vi "临界安全监督实测.vi"() -> ()   [LabVIEW 2020]
uses:
  <vilib>/Utility/sysdir.llb/System Directory Type.ctl
  <vilib>/Utility/error.llb/DialogType.ctl
  <vilib>/Utility/miscctls.llb/LVRowAndColumnTypeDef.ctl
  <vilib>/Analysis/baseanly.llb/Mean (DBL).vi
  GlobalVariable.vi
  <vilib>/Utility/inputDevices.llb/mouseAcquire.vi
  <vilib>/Analysis/NI_AALBase.lvlib
panel:
  in  "操作选项卡":enum32{"数据记录", "监督设置"}(tab)
  out "Table":string[][](table) caption="汇总表格"
  out "表象周期":sgl[](array[numeric])
  out "中子通量":sgl[](array[numeric])
  in  "保存表格":bool
  in  "添加记录":bool
  in  "显示临界曲线":bool
  in  "重设间隔":i32(knob)=1 min=1 max=100 step=1 scale=1.0..100.0
  in  "周期拟合个数":i32(knob)=1 min=1 max=100 step=1 scale=1.0..100.0
  out "堆芯参数：":dbl
  in  "堆芯参数项":u16(ring) items=["S棒位"]
  out "数选个数":i32
  in  "停止监督":bool
  in  "输入备注说明":string
  out "曲线5数字":dbl
  out "曲线4数字":dbl caption="D棒位"
  out "曲线3数字":dbl caption="电流2a周期"
  out "曲线2数字":dbl caption="电流2a"
  out "曲线1数字":dbl caption="电流1a周期"
  out "曲线0数字":dbl caption="电流1a"
  in  "自动/手动调整X标尺？":bool
  in  "X标尺最小-":bool
  in  "X标尺最小+":bool
  in  "自动调整Y标尺？":bool
  in  "Y标尺最小-":bool
  in  "Y标尺最小+":bool
  in  "Y标尺最大-":bool
  in  "Y标尺最大+":bool
  in  "曲线开关4":bool=TRUE
  in  "曲线开关5":bool=TRUE
  in  "曲线开关3":bool=TRUE
  in  "曲线开关2":bool=TRUE
  in  "曲线开关1":bool=TRUE
  in  "曲线开关0":bool=TRUE
  out "GraphChart":dbl[][](graph)
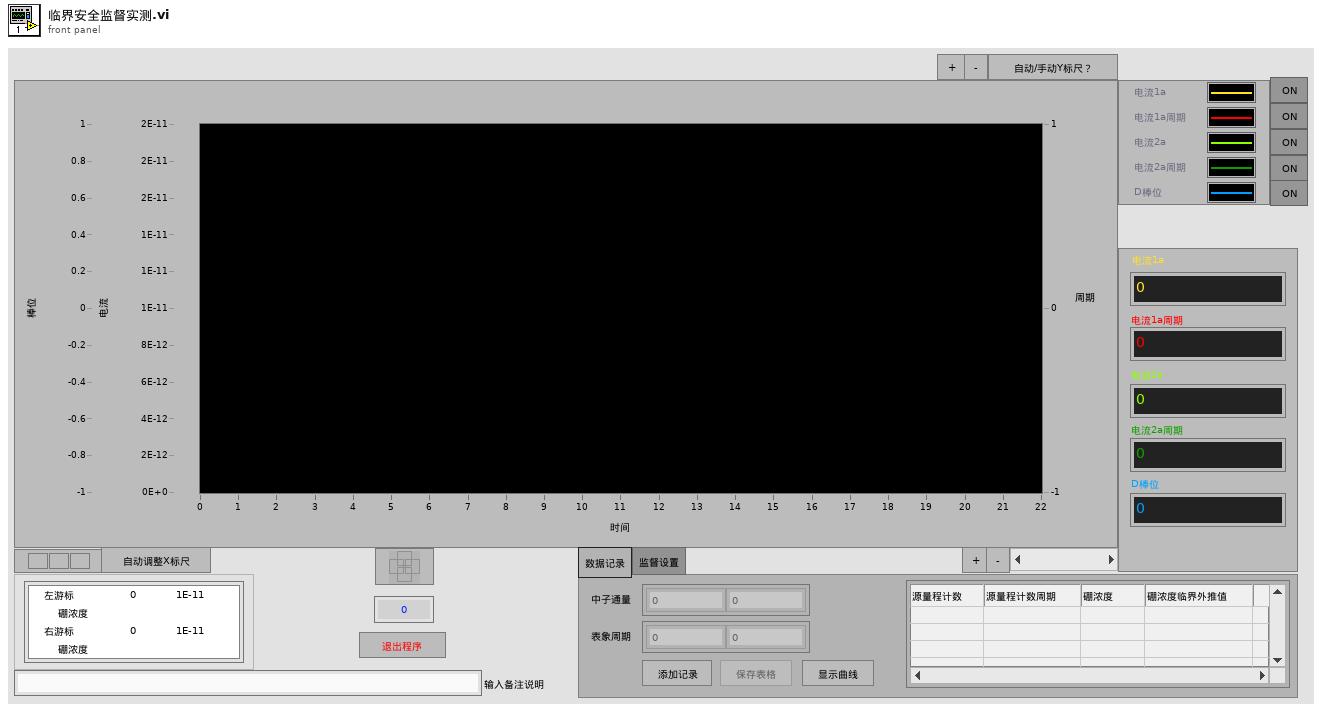
[diagram p1: front panel]
types:
  T1 = enum16{"open", "open or create", "create or replace", "create", "open (read only)"}
  T2 = typedef "System Directory Type.ctl" = i32
  T3 = typedef "DialogType.ctl" = u16
  T4 = enum8{"Enabled", "Disabled", "Disabled and Grayed Out"}
  T5 = enum16{"open", "replace", "create", "open or create", "replace or create", "replace or create with confirmation"}
  T6 = typedef "LVRowAndColumnTypeDef.ctl" = cluster{"Row":i32, "Column":i32}
  T7 = typedef "LVCursorListTypeDef.ctl" = cluster{"Name":string, "Color":u32, "Style":u8, "Point Style":u8, "Name Visible":bool, "Allow Drag":bool, "Cursor Mode":u32, "Plot":i32, "Index":i32, "Position":cluster{"X":dbl, "Y":dbl}, "X Scale":u32, "Y Scale":u32, "Watch Plots":i32[], "Watch All Plots":bool, "Plot Area":i32, "Label Offset":cluster{"X":dbl, "Y":dbl}}[]
  T8 = cluster{"Name":string, "Color":u32, "Style":u8, "Point Style":u8, "Name Visible":bool, "Allow Drag":bool, "Cursor Mode":u32, "Plot":i32, "Index":i32, "Position":cluster{"X":dbl, "Y":dbl}, "X Scale":u32, "Y Scale":u32, "Watch Plots":i32[], "Watch All Plots":bool, "Plot Area":i32, "Label Offset":cluster{"X":dbl, "Y":dbl}}
  T9 = cluster{"button 1":bool, "button 2":bool, "button 3":bool, "button 4":bool}
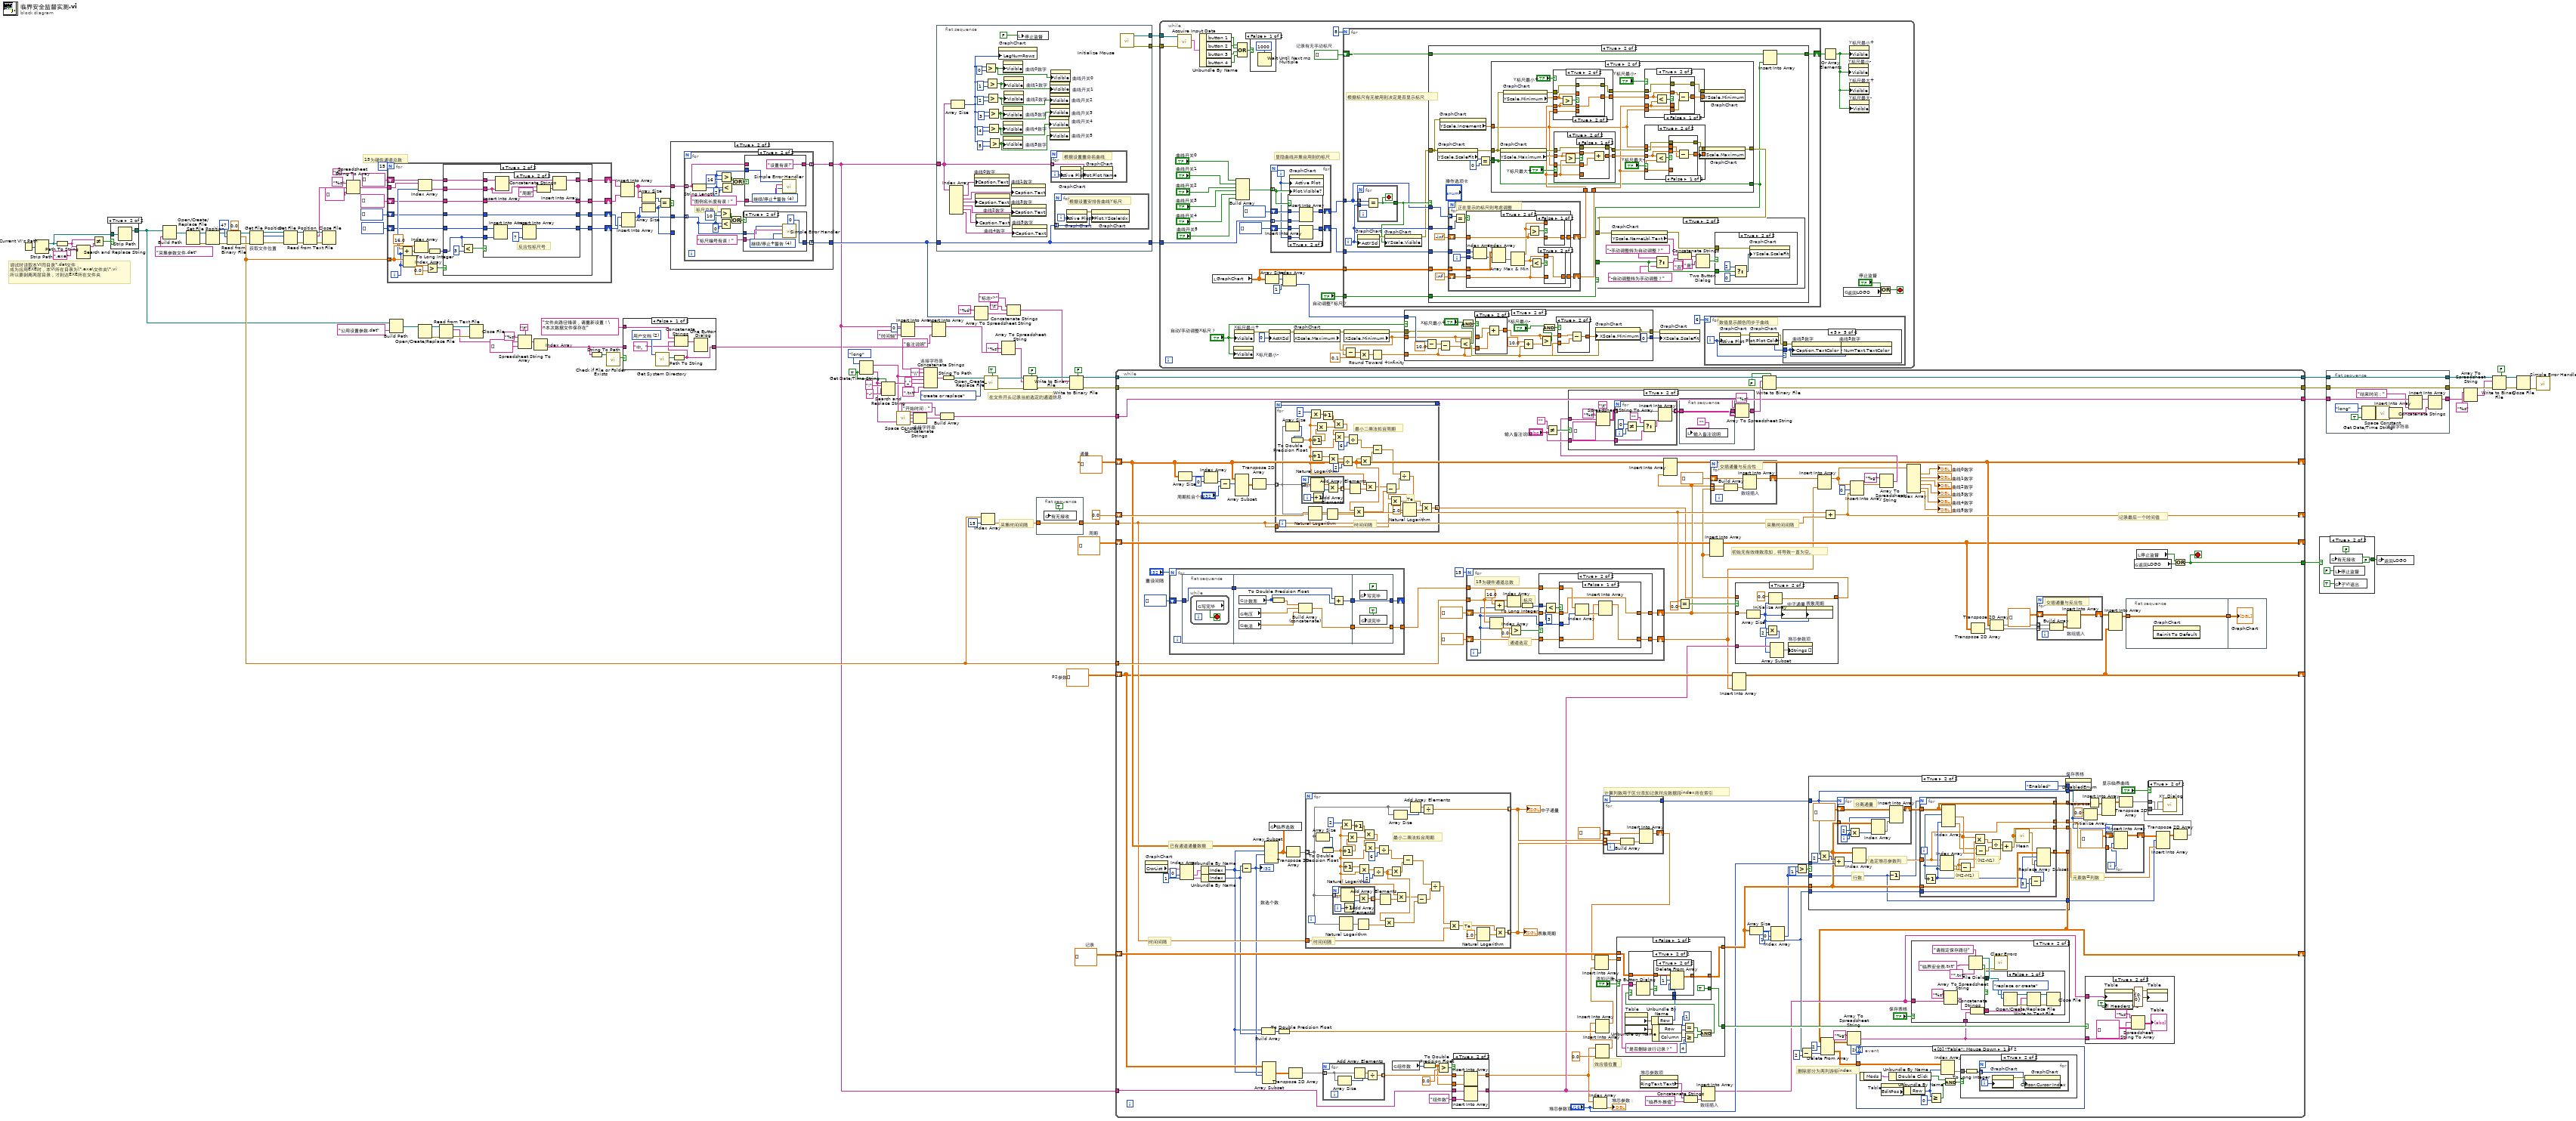
[diagram p0: block diagram]
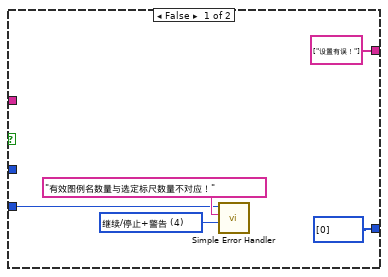
[diagram p4: hidden frame]
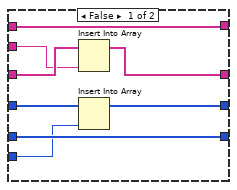
[diagram p8: hidden frame]
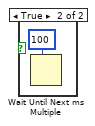
[diagram p9: hidden frame]
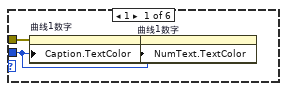
[diagram p10: hidden frame]
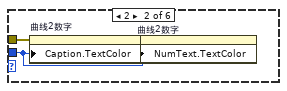
[diagram p11: hidden frame]
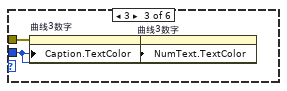
[diagram p12: hidden frame]
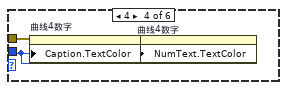
[diagram p13: hidden frame]
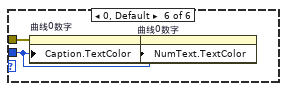
[diagram p14: hidden frame]
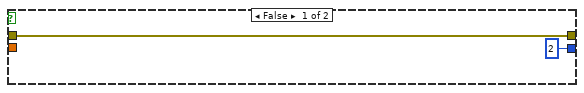
[diagram p15: hidden frame]
diagram:
  w22 = dbl[][] []  # P2参数
  w23 = dbl[][] []  # 周期
  w24 = dbl[][] []  # 通量
  w25 = dbl[][] []  # 记录
  w53 = TRUE ("需要秒？(F)")
  # "采集时间间隔"
  # "调试时读取本VI同目录*.dat文件，\n成为应用EXE时，本VI所在目录为\\*.exe\\文件夹\\*.vi\n所以要剥离两层目录，才到达EXE所在文件夹"
  # "15为硬件通道总数"
  # "在文件开头记录当前选定的通道信息"
  n1 = Current VI's Path() -> (path=w36:path)
  n2 = Strip Path(path=w36) -> (stripped path=w31:path)  [unwired: 1 out]
  n3 = Path To String(path=w31) -> (string=w33:string)
  n4 = Search and Replace String(input string=w33, search string=".exe" ("搜索字符串")) -> (result string=w34:string)  [unwired: 6 in, 3 out]
  n5 = Not Equal?(x=w33, y=w34) -> (x != y?=w32:bool)
  n6 = case shown="True" w32 {
    tunnel: w31 -> [w126 w128]
    tunnel: [w126 w127] -> w9
    frame False {
    }
    frame True {
      n7 = Strip Path(path=w128) -> (stripped path=w127:path)  [unwired: 1 out]
    }
  }
  n8 = Build Path(base path=w9, name or relative path="采集参数文件.dat") -> (appended path=w102:path)
  n9 = Open/Create/Replace File(file path (use dialog)=w102) -> (refnum out=w99:refnum<file>, error out=w98:errorcluster)  [unwired: 5 in, 1 out]
  n10 = Set File Position(refnum=w99, error in=w98) -> (refnum out=w97:refnum<file>, error out=w96:errorcluster)  [unwired: 2 in]
  n11 = Read from Binary File(5:sgl 0.0 ("byte stream type"), 8:w96, 10:47 ("count"), 11:w97) -> (0:w100:errorcluster, 2:w30:sgl[], 3:w101:refnum<file>)  [unwired: 2 in, 1 out]
  n12 = Get File Position "获取文件位置"(4:w100, 7:w101) -> (0:w104:errorcluster, 2:w91:i64, 3:w105:refnum<file>)
  n13 = Set File Position(offset (in bytes) (0)=w91, refnum=w105, error in=w104) -> (refnum out=w95:refnum<file>, error out=w94:errorcluster)  [unwired: 1 in]
  n14 = Read from Text File(file (use dialog)=w95, error in=w94) -> (refnum out=w92:refnum<file>, text=w87:string, error out=w93:errorcluster)  [unwired: 1 in, 2 out]
  n15 = Close File(refnum=w92, error in=w93) -> ()  [unwired: 2 out]
  n16 = Spreadsheet String To Array(delimiter (Tab)="\t", format string="%s", spreadsheet string=w87, array type (2D Dbl)=string[] [] ("添加的数组")) -> (array=w86:string[])
  n17 = for {
    N: 15 -> [_]
    tunnel: w30 -> [w140]
    tunnel: w86 -> [w147]
    shift-right: [w144] -> w80
    shift-left: string[] [] ("添加的数组") -> [w143]
    shift-right: [w135] -> w78
    shift-left: i32[] [] ("添加的数组") -> [w136]
    shift-right: [w133] -> w79
    shift-left: string[] [] ("添加的数组") -> [w134]
    shift-right: [w131] -> w77
    shift-left: i32[] [] ("添加的数组") -> [w132]
    i -> [w137]
    n18 = Add(x=16.0, y=w137) -> (x+y=w139:dbl)
    n19 = Index Array(array=w140, index=w137) -> (element=w146:sgl)
    n20 = Index Array(array=w140, index=w139) -> (element=w130:sgl)
    n21 = Index Array(array=w147, index=w137) -> (element=w141:string)
    n22 = Greater?(x=w146, y=sgl 0.0) -> (0:w142:bool)
    n23 = To Long Integer(number=w130) -> (32bit integer=w129:i32)
    n24 = case shown="True" w142 {
      tunnel: [w151 w163] -> w144
      tunnel: w143 -> [w151 w159]
      tunnel: w141 -> [_ w158]
      tunnel: [w150 w161] -> w135
      tunnel: w136 -> [w150 w153]
      tunnel: w134 -> [w149 w157]
      tunnel: [w149 w156] -> w133
      tunnel: w132 -> [w148 w155]
      tunnel: [w148 w154] -> w131
      tunnel: w129 -> [_ w152]
      frame False {
      }
      frame True {
        n25 = Less?(x=w152, y=3) -> (x < y?=w160:bool)
        n26 = case shown="True" w160 {
          tunnel: w159 -> [w170 w179]
          tunnel: [w170 w184] -> w163
          tunnel: w153 -> [w171 w174]
          tunnel: [w171 w183] -> w161
          tunnel: w158 -> [w167 w177]
          tunnel: w157 -> [w169 w176]
          tunnel: [w168 w176] -> w156
          tunnel: [w164 w175] -> w154
          tunnel: w155 -> [w166 w175]
          tunnel: w152 -> [w165 w172]
          frame False {
            n27 = Insert Into Array(array=w169, new element=w167) -> (w168:string[])  [unwired: 1 in]
            n28 = Insert Into Array(array=w166, new element=w165) -> (w164:i32[])  [unwired: 1 in]
          }
          frame True {
            # "反应性标尺号"
            n29 = Insert Into Array(array=w174, new element=w172) -> (w173:i32[])  [unwired: 1 in]
            n30 = Insert Into Array(array=w179, new element=w177) -> (w178:string[])  [unwired: 1 in]
            n31 = Insert Into Array(array=w173, new element=7 ("新元素/子数组")) -> (w183:i32[])  [unwired: 1 in]
            n32 = Concatenate Strings(w177, "周期" ("字符串")) -> (w181:string)
            n33 = Insert Into Array(array=w178, new element=w181) -> (w184:string[])  [unwired: 1 in]
          }
        }
      }
    }
  }
  n34 = Build Path(base path=w9, name or relative path="公用设置参数.dat") -> (appended path=w19:path)
  n35 = Open/Create/Replace File(file path (use dialog)=w19) -> (refnum out=w16:refnum<file>, error out=w15:errorcluster)  [unwired: 5 in, 1 out]
  n36 = Read from Text File(file (use dialog)=w16, error in=w15) -> (refnum out=w17:refnum<file>, text=w11:string, error out=w18:errorcluster)  [unwired: 1 in, 2 out]
  n37 = Close File(refnum=w17, error in=w18) -> ()  [unwired: 2 out]
  n38 = Spreadsheet String To Array(delimiter (Tab)="\t", format string="%s", spreadsheet string=w11, array type (2D Dbl)=string[] [] ("添加的数组")) -> (array=w10:string[])
  n39 = Index Array(array=w10) -> (element=w3:string)  [unwired: 1 in]
  n40 = String To Path(string=w3) -> (path=w5:path)
  n41 = call <vilib>:"Check if File or Folder Exists.vi"("path"=w5) -> ("file or folder exists?"=w4:bool)  [unwired: 8 in, 2 out]
  n42 = Insert Into Array(array=w80, new element=w79) -> (w72:string[])  [unwired: 1 in]
  n43 = Insert Into Array(array=w78, new element=w77) -> (w73:i32[])  [unwired: 1 in]
  n44 = case shown="False" w4 {
    tunnel: w3 -> [_ w191]
    tunnel: [w185 w191] -> w2
    tunnel: "文件夹路径错误，请重新设置！\n本次数据文件保存在" ("消息") -> [w189 _]
    frame False {
      w190 = T2 2 items=["用户目录"=0, "用户桌面"=1, "用户文档"=2, "用户应用程序数据"=3, "用户设置"=4, "用户临时目录"=5, "公共文档"=6, "公共应用程序数据"=7, "公共设置"=8, "公共缓存"=13, "系统核心库"=9, "系统安装库"=10, "应用程序文件"=11, "启动盘根目录"=12] ("system directory type")
      n45 = call <vilib>:"Get System Directory.vi"("system directory type"=w190) -> ("system directory"=w187:path)  [unwired: 10 in]
      n46 = Path To String(path=w187) -> (string=w185:string)
      n47 = Concatenate Strings(w189, w185, "中。" ("字符串")) -> (w188:string)
      n48 = One Button Dialog(message=w188) -> ()  [unwired: 1 in, 1 out]
    }
    frame True {
    }
  }
  n49 = Array Size(array=w72) -> (size(s)=w76:i32)
  n50 = Array Size(array=w73) -> (size(s)=w74:i32)
  n51 = Equal?(x=w76, y=w74) -> (x = y?=w75:bool)
  n52 = case shown="True" w75 {
    tunnel: w74 -> [w194 _]
    tunnel: w73 -> [_ w200]
    tunnel: w72 -> [_ w199]
    tunnel: [i32[] [0] w198] -> w63
    tunnel: [string[] ["设置有误！"] w197] -> w26
    frame False {
      w196 = T3 4 items=["无对话框", "确定信息", "继续或停止信息", "确定信息＋警告", "继续/停止+警告"] ("type of dialog (OK msg:1)")
      n53 = call <vilib>:"Simple Error Handler.vi"("error code (no error:0)"=w194, "error source (\" \")"="有效图例名数量与选定标尺数量不对应！" ("error source (\" \")"), "type of dialog (OK msg:1)"=w196) -> ()  [unwired: 2 in, 5 out]
    }
    frame True {
      n54 = for {
        tunnel: w200 -> [w205] mode=indexing
        tunnel: w199 -> [w202] mode=indexing
        tunnel: [w203] -> w198 mode=indexing
        tunnel: [w201] -> w197 mode=indexing
        # "标尺总数"
        n55 = String Length(string=w202) -> (length=w207:i32)
        n56 = Greater?(x=w205, y=10) -> (0:w210:bool)
        n57 = Less?(x=w205, y=0) -> (x < y?=w209:bool)
        n58 = Greater?(x=w207, y=16) -> (0:w214:bool)
        n59 = Less?(x=w207, y=2) -> (x < y?=w215:bool)
        n60 = Or(x=w210, y=w209) -> (x .or. y?=w206:bool)
        n61 = Or(x=w214, y=w215) -> (x .or. y?=w213:bool)
        n62 = case shown="True" w206 {
          tunnel: "标尺编号有误！" ("error source (\" \")") -> [_ w222]
          tunnel: w205 -> [w218 w221]
          tunnel: [w218 0] -> w203
          frame False {
          }
          frame True {
            w220 = T3 4 items=["无对话框", "确定信息", "继续或停止信息", "确定信息＋警告", "继续/停止+警告"] ("type of dialog (OK msg:1)")
            n63 = call <vilib>:"Simple Error Handler.vi"("error code (no error:0)"=w221, "error source (\" \")"=w222, "type of dialog (OK msg:1)"=w220) -> ()  [unwired: 2 in, 5 out]
          }
        }
        n64 = case shown="True" w213 {
          tunnel: "图例名长度有误！" ("error source (\" \")") -> [_ w227]
          tunnel: w207 -> [_ w226]
          tunnel: w202 -> [w223 _]
          tunnel: [w223 "设置有误!"] -> w201
          frame False {
          }
          frame True {
            w225 = T3 4 items=["无对话框", "确定信息", "继续或停止信息", "确定信息＋警告", "继续/停止+警告"] ("type of dialog (OK msg:1)")
            n65 = call <vilib>:"Simple Error Handler.vi"("error code (no error:0)"=w226, "error source (\" \")"=w227, "type of dialog (OK msg:1)"=w225) -> ()  [unwired: 2 in, 5 out]
          }
        }
      }
    }
  }
  n66 = Get Date/Time String(date format (0)=enum16{"short", "long", "abbreviated"}."long" ("日期格式(0)"), want seconds? (F)=w53) -> (date string=w51:string, time string=w50:string)  [unwired: 1 in]
  n67 = Search and Replace String(replace all?=w53, input string=w50, search string=":", replace string="-" ("replace string (\"\")")) -> (result string=w121:string)  [unwired: 4 in, 3 out]
  n68 = call <vilib>:"Space Constant.vi"() -> ("String"=w52:string)
  n69 = Insert Into Array(array=w26, index=0 ("索引"), new element="时间轴" ("新元素/子数组")) -> (w57:string[])
  n70 = Concatenate Strings "连接字符串"(w51, w52, w50) -> (w47:string)
  n71 = Concatenate Strings "连接字符串"(w2, "\\" ("字符串"), w51, "_" ("string"), w121, ".txt" ("string")) -> (w7:string)
  n72 = Insert Into Array(array=w57, new element="备注说明" ("新元素/子数组")) -> (w56:string[])  [unwired: 1 in]
  n73 = flat-sequence {
    tunnel: w26 -> [w239]
    tunnel: [w229] -> w111
    tunnel: w63 -> [w229]
    tunnel: [w231] -> w109
    tunnel: [w230] -> w108
    frame #0 {
      n74 = Index Array(array=w239) -> (element #1=w251:string, element #2=w250:string, element #3=w249:string, element #4=w248:string, element #5=w247:string, element #6=w246:string)  [unwired: 6 in]
      n75 = Array Size(array=w239) -> (size(s)=w232:i32)
      n76 = property on="曲线0数字" class="DigNum (strict)"("Caption.Text"=w251) -> ()  [unwired: 2 in, 2 out]
      n77 = property on="曲线2数字" class="DigNum (strict)"("Caption.Text"=w249) -> ()  [unwired: 2 in, 2 out]
      n78 = property on="曲线4数字" class="DigNum (strict)"("Caption.Text"=w247) -> ()  [unwired: 2 in, 2 out]
      n79 = Greater?(x=w232, y=0) -> (0:w238:bool)
      n80 = Greater?(x=w232, y=1) -> (0:w237:bool)
      n81 = Greater?(x=w232, y=2) -> (0:w236:bool)
      n82 = Greater?(x=w232, y=3) -> (0:w235:bool)
      n83 = Greater?(x=w232, y=4) -> (0:w234:bool)
      n84 = Greater?(x=w232, y=5) -> (0:w233:bool)
      n85 = property on="GraphChart" class="WFGraph (strict)"("LegNumRows"=w232) -> ()  [unwired: 2 in, 2 out]
      n86 = property on="曲线0数字" class="DigNum (strict)"("Visible"=w238) -> ()  [unwired: 2 in, 2 out]
      n87 = property on="曲线3数字" class="DigNum (strict)"("Visible"=w235) -> ()  [unwired: 2 in, 2 out]
      n88 = property on="曲线4数字" class="DigNum (strict)"("Visible"=w234) -> ()  [unwired: 2 in, 2 out]
      n89 = property on="曲线5数字" class="DigNum (strict)"("Visible"=w233) -> ()  [unwired: 2 in, 2 out]
      n90 = property on="曲线1数字" class="DigNum (strict)"("Visible"=w237) -> ()  [unwired: 2 in, 2 out]
      n91 = property on="曲线2数字" class="DigNum (strict)"("Visible"=w236) -> ()  [unwired: 2 in, 2 out]
      n92 = property on="曲线1数字" class="DigNum (strict)"("Caption.Text"=w250) -> ()  [unwired: 2 in, 2 out]
      n93 = property on="曲线3数字" class="DigNum (strict)"("Caption.Text"=w248) -> ()  [unwired: 2 in, 2 out]
      n94 = property on="曲线5数字" class="DigNum (strict)"("Caption.Text"=w246) -> ()  [unwired: 2 in, 2 out]
      n95 = local write "停止监督"(FALSE ("stop")) -> ()
      n96 = property on="曲线开关4" class="Bool (strict)"("Visible"=w234) -> ()  [unwired: 2 in, 2 out]
      n97 = property on="曲线开关2" class="Bool (strict)"("Visible"=w236) -> ()  [unwired: 2 in, 2 out]
      n98 = property on="曲线开关3" class="Bool (strict)"("Visible"=w235) -> ()  [unwired: 2 in, 2 out]
      n99 = property on="曲线开关5" class="Bool (strict)"("Visible"=w233) -> ()  [unwired: 2 in, 2 out]
      n100 = property on="曲线开关1" class="Bool (strict)"("Visible"=w237) -> ()  [unwired: 2 in, 2 out]
      n101 = property on="曲线开关0" class="Bool (strict)"("Visible"=w238) -> ()  [unwired: 2 in, 2 out]
      n102 = for {
        tunnel: w239 -> [w256] mode=indexing
        i -> [w257]
        # "根据设置重命名曲线"
        n103 = property on="GraphChart" class="WFGraph (strict)"("Active Plot"=w257) -> (error out=w255:errorcluster)  [unwired: 2 in, 1 out]
        n104 = property on="GraphChart" class="WFGraph (strict)"(error in=w255, "Plot.Plot Name"=w256) -> ()  [unwired: 1 in, 2 out]
      }
      n105 = for {
        tunnel: w229 -> [w252] mode=indexing
        i -> [w254]
        # "根据设置安排各曲线Y标尺"
        n106 = property on="GraphChart" class="WFGraph (strict)"("Active Plot"=w254) -> (error out=w253:errorcluster)  [unwired: 2 in, 1 out]
        n107 = property on="GraphChart" class="WFGraph (strict)"(error in=w253, "Plot.YScaleIdx"=w252) -> ()  [unwired: 1 in, 2 out]
      }
      n108 = call <vilib>:"Initialize Mouse.vi"() -> ("error out"=w231:errorcluster, "device ID"=w230:refnum<k1>)  [unwired: 1 in, 9 out]
    }
  }
  n109 = Build Array("开始时间：" ("字符串"), w47) -> (w45:string[])
  n110 = String To Path(string=w7) -> (path=w6:path)
  n111 = Array To Spreadsheet String(array=w63, 3:"%d" ("format string")) -> (spreadsheet string=w62:string)  [unwired: 1 in]
  n112 = Index Array(array=w30, index=15 ("索引")) -> (element=w28:sgl)
  n113 = call <vilib>:"Open_Create_Replace File.vi"("advisory dialog? (display:T)"=TRUE, "function (open:0)"=T1."create or replace", "file path"=w6) -> ("error out"=w118:errorcluster, "refnum"=w114:refnum<file>)  [unwired: 5 in, 2 out]
  n114 = Array To Spreadsheet String(array=w56, 3:"%s" ("format string")) -> (spreadsheet string=w110:string)  [unwired: 1 in]
  n115 = Concatenate Strings("标志->" ("字符串"), "\t", w62) -> (w59:string)
  n116 = Write to Binary File(file (use dialog)=w114, data=w110, error in=w118, 5:FALSE ("预置数组或字符串大小？(T)")) -> (refnum out=w67:refnum<file>, error out=w66:errorcluster)  [unwired: 2 in, 1 out]
  n117 = flat-sequence {
    tunnel: w28 -> [w258]
    tunnel: [w258] -> w27
    frame #0 {
      n118 = global write "GlobalVariable.vi" "有无接收"(TRUE ("写完毕")) -> ()
    }
  }
  n119 = Write to Binary File(file (use dialog)=w67, data=w59, error in=w66, 5:FALSE ("预置数组或字符串大小？(T)")) -> (refnum out=w65:refnum<file>, error out=w64:errorcluster)  [unwired: 2 in, 1 out]
  n120 = while {
    shift-right: [w310] -> _
    shift-left: w24 -> [w313]
    tunnel: w65 -> [w392]
    tunnel: w64 -> [w395]
    tunnel: [w264] -> w119
    tunnel: [w394] -> w116
    tunnel: [w391] -> w112
    tunnel: w30 -> [w382]
    shift-right: [w314] -> _
    shift-left: 0.0 -> [w325]
    tunnel: w45 -> [w372]
    tunnel: [w372] -> w49
    tunnel: w27 -> [w303]
    tunnel: w26 -> [w294]
    shift-right: [w280] -> _
    shift-left: w25 -> [w370]
    shift-right: [w308] -> _
    shift-left: w23 -> [w318]
    shift-right: [w328] -> _
    shift-left: w22 -> [w298]
    stop <- w264 stop-if-true
    # "元素数=列数"
    # "删除部分为两列游标index"
    # "时间间隔"
    # "初始无有效维数添加，将导致一直为空。"
    # "效应值位置"
    # "计算列数用于区分添加记录对应数据段index所在索引"
    # "已有通道通量数据"
    # "记录最后一个时间值"
    # "采集时间间隔"
    n121 = property on="GraphChart" class="WFGraph (strict)"() -> ("CrsrList"=w331:T7)  [unwired: 2 in, 2 out]
    n122 = for {
      N: "重设间隔" -> [_]
      shift-right: [w636] -> _
      shift-left: u32[] [] ("data") -> [w639]
      tunnel: [w634] -> w263
      n123 = flat-sequence {
        tunnel: [w640] -> w638
        tunnel: w639 -> [w640]
        tunnel: w638 -> [w647]
        tunnel: [w648] -> w637
        tunnel: [w644] -> w635
        tunnel: [w651] -> w636
        tunnel: w637 -> [w651]
        tunnel: w635 -> [w649]
        tunnel: [w649] -> w634
        frame #0 {
          n124 = while {
            stop <- w641 stop-if-true
            n125 = global read "GlobalVariable.vi" "写完毕"() -> (w641:bool)
          }
        }
        frame #1 {
          n126 = global read "GlobalVariable.vi" "计数率"() -> (w646:u32[])
          n127 = global read "GlobalVariable.vi" "电压"() -> (w643:dbl[])
          n128 = global read "GlobalVariable.vi" "电流"() -> (w642:dbl[])
          n129 = To Double Precision Float(number=w646) -> (double precision float=w645:dbl[])
          n130 = Build Array (concatenate)(w645, w643, w642) -> (w644:dbl[])
          n131 = Add(x=w647, y=w646) -> (x+y=w648:u32[])
        }
        frame #2 {
          n132 = global write "GlobalVariable.vi" "写完毕"(FALSE ("写完毕")) -> ()
          n133 = global write "GlobalVariable.vi" "读完毕"(TRUE ("写完毕")) -> ()
        }
      }
    }
    n134 = Array Size(array=w313) -> (size(s)=w322:i32[])
    n135 = Index Array(array=w331, index #1=0 ("index"), index #2=1 ("index")) -> (element #1=w367:T8, element #2=w369:T8)
    n136 = Unbundle By Name(w367) -> ("Index"=w286:i32)
    n137 = Unbundle By Name(w369) -> ("Index"=w302:i32)
    n138 = Index Array(array=w322, index=0 ("索引")) -> (element=w320:i32)
    n139 = Subtract(x=w320, y="周期拟合个数") -> (x-y=w306:i32)
    n140 = Array Subset(array=w313, index (row)=w306) -> (w305:dbl[][])  [unwired: 3 in]
    n141 = Subtract(x=w302, y=w286) -> (x-y=w287:i32)
    "数选个数" <- w287
    n142 = Transpose 2D Array(2D array=w305) -> (transposed array=w304:dbl[][])
    n143 = Build Array(w286, w302) -> (w356:i32[])
    n144 = Array Subset(array=w298, index (row)=w286, length (row)=w287) -> (w300:dbl[][])  [unwired: 2 in]
    n145 = Array Subset(array=w313, index (row)=w286, length (row)=w287) -> (w297:dbl[][])  [unwired: 2 in]
    n146 = global write "GlobalVariable.vi" "临界选数"(w297) -> ()
    n147 = for {
      N -> [w413]
      tunnel: w304 -> [w414] mode=indexing
      tunnel: [w412] -> w317 mode=indexing
      tunnel: w303 -> [w443]
      tunnel: [w413] -> _
      # "时间间隔"
      # "最小二乘法拟合周期"
      # "Te"
      n148 = Array Size(array=w414) -> (size(s)=w419:i32)
      n149 = To Double Precision Float(number=w419) -> (double precision float=w418:dbl)
      n150 = for {
        tunnel: w414 -> [w448] mode=indexing
        tunnel: [w444] -> w432 mode=indexing
        i -> [w447]
        n151 = Natural Logarithm(1:w448) -> (0:w446:dbl)
        n152 = Increment(x=w447) -> (x+1=w445:i32)
        n153 = Multiply(x=w446, y=w445) -> (x*y=w444:dbl)
      }
      n154 = Natural Logarithm(1:w414) -> (0:w427:dbl[])
      n155 = Multiply(x=2 ("count"), y=w418) -> (x*y=w439:dbl)
      n156 = Increment(x=w418) -> (x+1=w442:dbl)
      n157 = Increment(x=w418) -> (x+1=w436:dbl)
      n158 = Multiply(x=w418, y=w442) -> (x*y=w440:dbl)
      n159 = Increment(x=w439) -> (x+1=w438:dbl)
      n160 = Add Array Elements(numeric array=w427) -> (sum=w426:dbl)
      n161 = Multiply(x=w436, y=w418) -> (x*y=w435:dbl)
      n162 = Multiply(x=w438, y=w440) -> (x*y=w437:dbl)
      n163 = Multiply(x=w437, y=w418) -> (x*y=w422:dbl)
      n164 = Divide(x=w435, y=2 ("count")) -> (x/y=w430:dbl)
      n165 = Divide(x=w422, y=6 ("count")) -> (x/y=w420:dbl)
      n166 = Add Array Elements(numeric array=w432) -> (sum=w433:dbl)
      n167 = Multiply(x=w430, y=w426) -> (x*y=w428:dbl)
      n168 = Multiply(x=w430, y=w430) -> (x*y=w431:dbl)
      n169 = Multiply(x=w418, y=w433) -> (x*y=w429:dbl)
      n170 = Subtract(x=w420, y=w431) -> (x-y=w424:dbl)
      n171 = Subtract(x=w429, y=w428) -> (x-y=w425:dbl)
      n172 = Divide(x=w424, y=w425) -> (x/y=w423:dbl)
      n173 = Multiply(x=w423, y=w443) -> (x*y=w415:dbl)
      n174 = Natural Logarithm(1:sgl 2.0) -> (0:w417:sgl)
      n175 = Multiply(x=w415, y=w417) -> (x*y=w412:dbl)
    }
    n176 = To Double Precision Float(number=w356) -> (double precision float=w352:dbl[])
    n177 = Transpose 2D Array(2D array=w297) -> (transposed array=w301:dbl[][])
    n178 = Transpose 2D Array(2D array=w300) -> (transposed array=w299:dbl[][])
    n179 = for {
      tunnel: w301 -> [w595] mode=indexing
      tunnel: [w627] -> w327 mode=indexing
      tunnel: w303 -> [w628]
      tunnel: [w596] -> w326 mode=indexing
      # "时间间隔"
      # "最小二乘法拟合周期"
      # "Te"
      n180 = Array Size(array=w595) -> (size(s)=w603:i32)
      n181 = To Double Precision Float(number=w603) -> (double precision float=w602:dbl)
      n182 = for {
        tunnel: w595 -> [w633] mode=indexing
        tunnel: [w629] -> w616 mode=indexing
        i -> [w632]
        n183 = Natural Logarithm(1:w633) -> (0:w631:dbl)
        n184 = Increment(x=w632) -> (x+1=w630:i32)
        n185 = Multiply(x=w631, y=w630) -> (x*y=w629:dbl)
      }
      n186 = Natural Logarithm(1:w595) -> (0:w611:dbl[])
      n187 = Multiply(x=2 ("count"), y=w602) -> (x*y=w623:dbl)
      n188 = Increment(x=w602) -> (x+1=w626:dbl)
      n189 = Increment(x=w602) -> (x+1=w620:dbl)
      n190 = Multiply(x=w602, y=w626) -> (x*y=w624:dbl)
      n191 = Increment(x=w623) -> (x+1=w622:dbl)
      n192 = Add Array Elements(numeric array=w611) -> (sum=w610:dbl)
      n193 = Multiply(x=w620, y=w602) -> (x*y=w619:dbl)
      n194 = Multiply(x=w622, y=w624) -> (x*y=w621:dbl)
      n195 = Multiply(x=w621, y=w602) -> (x*y=w606:dbl)
      n196 = Divide(x=w619, y=2 ("count")) -> (x/y=w614:dbl)
      n197 = Divide(x=w606, y=6 ("count")) -> (x/y=w604:dbl)
      n198 = Add Array Elements(numeric array=w616) -> (sum=w617:dbl)
      n199 = Multiply(x=w614, y=w610) -> (x*y=w612:dbl)
      n200 = Multiply(x=w614, y=w614) -> (x*y=w615:dbl)
      n201 = Array Size(array=w595) -> (size(s)=w597:i32)
      n202 = Multiply(x=w602, y=w617) -> (x*y=w613:dbl)
      n203 = Subtract(x=w604, y=w615) -> (x-y=w608:dbl)
      n204 = Add Array Elements(numeric array=w595) -> (sum=w598:dbl)
      n205 = Subtract(x=w613, y=w612) -> (x-y=w609:dbl)
      n206 = Divide(x=w598, y=w597) -> (x/y=w596:dbl)
      n207 = Divide(x=w608, y=w609) -> (x/y=w607:dbl)
      n208 = Multiply(x=w607, y=w628) -> (x*y=w599:dbl)
      n209 = Natural Logarithm(1:sgl 2.0) -> (0:w601:sgl)
      n210 = Multiply(x=w599, y=w601) -> (x*y=w627:dbl)
    }
    "表象周期" <- w327
    "中子通量" <- w326
    n211 = for {
      tunnel: w299 -> [w515] mode=indexing
      tunnel: [w514] -> w292 mode=indexing
      n212 = Array Size(array=w515) -> (size(s)=w516:i32)
      n213 = Add Array Elements(numeric array=w515) -> (sum=w517:dbl)
      n214 = Divide(x=w517, y=w516) -> (x/y=w514:dbl)
    }
    n215 = global read "GlobalVariable.vi" "组件数"() -> (w296:i32)
    n216 = To Double Precision Float(number=w296) -> (double precision float=w288:dbl)
    n217 = Greater?(x=w288, y=0.0) -> (0:w290:bool)
    n218 = case shown="True" w290 {
      tunnel: w294 -> [w404 w411]
      tunnel: [w404 w410] -> w293
      tunnel: w292 -> [w405 w409]
      tunnel: [w405 w408] -> w291
      tunnel: "组件数" ("新元素/子数组") -> [_ w407]
      tunnel: w288 -> [_ w406]
      frame False {
      }
      frame True {
        n219 = Insert Into Array(array=w409, new element=w406) -> (w408:dbl[])  [unwired: 1 in]
        n220 = Insert Into Array(array=w411, new element=w407) -> (w410:string[])  [unwired: 1 in]
      }
    }
    n221 = for {
      N: 15 -> [_]
      tunnel: w382 -> [w682]
      shift-right: [w678] -> w312
      shift-left: dbl[] [] ("data") -> [w679]
      shift-right: [w676] -> w267
      shift-left: dbl[] [] ("data") -> [w677]
      tunnel: w263 -> [w675]
      i -> [w674]
      # "15为硬件通道总数"
      # "标尺"
      # "通道选定"
      n222 = Index Array(array=w682, index=w674) -> (element=w687:sgl)
      n223 = Add(x=16.0, y=w674) -> (x+y=w685:dbl)
      n224 = Index Array(array=w682, index=w685) -> (element=w683:sgl)
      n225 = Greater?(x=w687, y=sgl 0.0) -> (0:w681:bool)
      n226 = To Long Integer(number=w683) -> (32bit integer=w680:i32)
      n227 = case shown="True" w681 {
        tunnel: w680 -> [_ w697]
        tunnel: w679 -> [w689 w695]
        tunnel: [w689 w694] -> w678
        tunnel: w677 -> [w688 w693]
        tunnel: [w688 w692] -> w676
        tunnel: w675 -> [_ w691]
        tunnel: w674 -> [_ w690]
        frame False {
        }
        frame True {
          n228 = Less?(x=w697, y=3) -> (x < y?=w696:bool)
          n229 = case shown="False" w696 {
            tunnel: w695 -> [w699 w707]
            tunnel: [w699 w705] -> w694
            tunnel: w693 -> [w703 w710]
            tunnel: [w700 w710] -> w692
            tunnel: w691 -> [w702 w709]
            tunnel: w690 -> [w701 w708]
            frame False {
              n230 = Index Array(array=w702, index=w701) -> (element=w704:dbl)
              n231 = Insert Into Array(array=w703, new element=w704) -> (w700:dbl[])  [unwired: 1 in]
            }
            frame True {
              n232 = Index Array(array=w709, index=w708) -> (element=w706:dbl)
              n233 = Insert Into Array(array=w707, new element=w706) -> (w705:dbl[])  [unwired: 1 in]
            }
          }
        }
      }
    }
    n234 = Not Equal?(x="", y="输入备注说明") -> (x != y?=w375:bool)
    n235 = Index Array(array=w291, index="堆芯参数项") -> (element=→"堆芯参数：":dbl)
    n236 = Insert Into Array(array=w291, new element=0.0 ("新元素/子数组")) -> (w344:dbl[])  [unwired: 1 in]
    n237 = Insert Into Array(array=w344, new element=w352) -> (w351:dbl[])  [unwired: 1 in]
    n238 = for {
      N -> [w589]
      tunnel: w326 -> [w594] mode=indexing
      tunnel: w327 -> [w593] mode=indexing
      shift-right: [w590] -> w359
      shift-left: dbl[] [] -> [w592]
      tunnel: [w589] -> w339
      n239 = Build Array(w594, w593) -> (w591:dbl[])
      n240 = Insert Into Array(array=w592, new element=w591) -> (w590:dbl[])  [unwired: 1 in]
    }
    n241 = Insert Into Array(array=w359, new element=w351) -> (w353:dbl[])  [unwired: 1 in]
    n242 = case shown="False" "添加记录" {
      tunnel: w370 -> [w564 w588]
      tunnel: w353 -> [_ w587]
      tunnel: [w563 w586] -> w343
      tunnel: [w562 TRUE] -> w363
      frame False {
        n243 = property on="Table" class="Tbl (strict)"() -> ("Selection Start"=w571:T6, "Selection Size"=w570:T6)  [unwired: 2 in, 2 out]
        n244 = Unbundle By Name(w571) -> ("Row"=w561:i32)
        n245 = Unbundle By Name(w570) -> ("Row"=w568:i32, "Column"=w558:i32)
        n246 = Equal?(x=1, y=w568) -> (x = y?=w560:bool)
        n247 = Greater Or Equal?(x=w558, y=4) -> (x >= y?=w559:bool)
        n248 = And(x=w560, y=w559) -> (x .and. y?=w566:bool)
        n249 = case shown="True" w566 {
          tunnel: "是否删除该行记录？" ("消息") -> [_ w579]
          tunnel: w561 -> [_ w577]
          tunnel: w564 -> [w573 w576]
          tunnel: [w573 w575] -> w563
          tunnel: [FALSE TRUE] -> w562
          frame False {
          }
          frame True {
            n250 = Two Button Dialog(message=w579) -> (T button?=w578:bool)  [unwired: 2 in]
            n251 = case shown="True" w578 {
              tunnel: w577 -> [_ w584]
              tunnel: w576 -> [w580 w583]
              tunnel: [w580 w581] -> w575
              frame False {
              }
              frame True {
                n252 = Delete From Array(array=w583, length=1 ("长度"), index (row)=w584) -> (array with subset deleted=w581:dbl[][])  [unwired: 1 in, 1 out]
              }
            }
          }
        }
      }
      frame True {
        n253 = Insert Into Array(array=w588, new element=w587) -> (w586:dbl[][])  [unwired: 2 in]
      }
    }
    n254 = property on="堆芯参数项" class="Ring (strict)"() -> ("RingText.Text"=w333:string)  [unwired: 2 in, 2 out]
    n255 = Insert Into Array(array=w313, new element=w312) -> (w310:dbl[][])  [unwired: 2 in]
    n256 = Equal?(x=w325, y=0.0) -> (x = y?=w323:bool)
    n257 = Concatenate Strings(w333, "临界外推值" ("新元素/子数组")) -> (w335:string)
    n258 = Insert Into Array "数组插入"(array=w293, new element=w335) -> (w285:string[])  [unwired: 1 in]
    n259 = Insert Into Array(array=w298, new element=w267) -> (w328:dbl[][])  [unwired: 2 in]
    n260 = case shown="True" w323 {
      tunnel: w312 -> [_ w457]
      tunnel: w317 -> [w449 _]
      tunnel: [w449 w456] -> w316
      tunnel: w293 -> [_ w454]
      frame False {
      }
      frame True {
        n261 = Array Size(array=w457) -> (size(s)=w453:i32)
        n262 = Multiply(x=w453, y=2) -> (x*y=w451:i32)
        n263 = Initialize Array(0.0 ("元素"), w453) -> (w456:dbl[])
        n264 = Array Subset ("数组子集")(array=w454, index=w451) -> (w450:string[])  [unwired: 1 in]
        n265 = property on="中子通量" class="Arr (strict)"("Number of Columns"=w453) -> (error out=w458:errorcluster)  [unwired: 2 in, 1 out]
        n266 = property on="堆芯参数项" class="Ring (strict)"("Strings []"=w450) -> ()  [unwired: 2 in, 2 out]
        n267 = property on="表象周期" class="Arr (strict)"(error in=w458, "Number of Columns"=w453) -> ()  [unwired: 1 in, 2 out]
      }
    }
    n268 = Insert Into Array ("数组插入")(array=w318, new element=w316) -> (w308:dbl[][])  [unwired: 2 in]
    n269 = for {
      tunnel: w312 -> [w711] mode=indexing
      tunnel: w316 -> [w712] mode=indexing
      shift-right: [w713] -> w268
      shift-left: dbl[] [] -> [w715]
      # "交插通量与反应性"
      n270 = Build Array(w711, w712) -> (w714:dbl[])
      n271 = Insert Into Array "数组插入"(array=w715, new element=w714) -> (w713:dbl[])  [unwired: 1 in]
    }
    n272 = Array Size(array=w343) -> (size(s)=w349:i32[])
    n273 = Index Array(array=w349, index #1=0 ("索引"), index #2=1 ("索引")) -> (element #1=w337:i32, element #2=w336:i32)
    n274 = Greater?(x=w337, y=1) -> (0:w346:bool)
    n275 = Subtract(x=w336, y=2) -> (x-y=w342:i32)
    n276 = case shown="True" w346 {
      tunnel: w343 -> [w470 w480]
      tunnel: w339 -> [_ w472]
      tunnel: "堆芯参数项" -> [_ w485]
      tunnel: w337 -> [_ w471]
      tunnel: [w470 w478] -> w280
      tunnel: w336 -> [_ w477]
      tunnel: [T4."Disabled and Grayed Out" ("禁用") T4."Enabled" ("禁用")] -> w332
      tunnel: [dbl[][] [] ("type (empty)") w475] -> w284
      tunnel: [dbl[] [] ("记录") w474] -> w278
      tunnel: [dbl[] [] w473] -> w273
      tunnel: [0 w472] -> w277
      tunnel: [0 w471] -> w272
      frame False {
      }
      frame True {
        # "行数"
        # "选定堆芯参数列"
        n277 = Multiply(x=w472, y=2) -> (x*y=w483:i32)
        n278 = Add(x=w483, y=w485) -> (x+y=w486:i32)
        n279 = for {
          N: w472 -> [_]
          tunnel: w480 -> [w513]
          shift-right: [w510] -> w482
          shift-left: dbl[][] [] ("type (empty)") -> [w511]
          i -> [w507]
          # "分离通量"
          n280 = Multiply(x=2 ("y"), y=w507) -> (x*y=w508:i32)
          n281 = Index Array(array=w513, index (col)=w508) -> (element=w509:dbl[])  [unwired: 1 in]
          n282 = Insert Into Array(array=w511, index (col)=w507, new element=w509) -> (w510:dbl[][])  [unwired: 1 in]
        }
        n283 = Index Array(array=w480, index (col)=w486) -> (element=w481:dbl[])  [unwired: 1 in]
        n284 = Decrement(x=w471) -> (x-1=w479:i32)
        n285 = for {
          N: w479 -> [_]
          tunnel: w482 -> [w489]
          tunnel: w481 -> [w488]
          tunnel: w480 -> [w503]
          tunnel: w477 -> [w505]
          tunnel: [w501] -> w478
          tunnel: [w490] -> w473
          tunnel: [w489] -> w475
          tunnel: [w488] -> w474
          i -> [w500]
          # "(N2-N1)"
          # "(M2-M1)"
          n286 = Increment(x=w500) -> (x+1=w499:i32)
          n287 = Index Array(array=w488, index #1=w500, index #2=w499) -> (element #1=w506:dbl, element #2=w492:dbl)
          n288 = Index Array(array=w489, index (row) #1=w500, index (row) #2=w499) -> (element #1=w497:dbl[], element #2=w494:dbl[])  [unwired: 2 in]
          n289 = Subtract(x=w492, y=w506) -> (x-y=w498:dbl)
          n290 = Multiply(x=w497, y=w498) -> (x*y=w496:dbl[])
          n291 = Subtract(x=w494, y=w497) -> (x-y=w495:dbl[])
          n292 = Divide(x=w496, y=w495) -> (x/y=w493:dbl[])
          n293 = Add(x=w493, y=w492) -> (x+y=w490:dbl[])
          n294 = call-poly <vilib>:"Mean.vi"("X"=w490) -> ("mean"=w491:dbl)  [unwired: 1 out]
          n295 = Subtract(x=w505, y=3) -> (x-y=w502:i32)
          n296 = Replace Array Subset(array=w503, new element=w491, index (row)=w499, index (col)=w502) -> (w501:dbl[][])
        }
      }
    }
    n297 = Insert Into Array(array=w268, new element=w267) -> (w262:dbl[])  [unwired: 1 in]
    n298 = Delete From Array(array=w280, length=2 ("长度"), index (col)=w342) -> (deleted portion=w355:dbl[][], array with subset deleted=w358:dbl[][])  [unwired: 1 in]
    n299 = Add(x=w325, y=w303) -> (x+y=w314:dbl)
    n300 = Array To Spreadsheet String(array=w358, 3:"%g" ("格式字符串")) -> (spreadsheet string=w361:string)  [unwired: 1 in]
    n301 = Insert Into Array(array=w262, index=0 ("索引 (行)"), new element=w314) -> (w315:dbl[])
    n302 = event shown="[0] \"Table\": Mouse Down" {
      selector: _ -> [_ _]
      dyn-events: _ -> [_ _]
      timeout: 20 -> [_ _]
      tunnel: w355 -> [w519 _]
      event "Table": Mouse Down {
        n303 = event-data() -> ("Mods"=w526:cluster{"Double Click":bool, "Menu Key":bool})  [unwired: 1 in]
        n304 = property on="Table" class="Tbl (strict)"() -> ("EditPos"=w524:T6)  [unwired: 2 in, 2 out]
        n305 = Unbundle By Name(w526) -> ("Double Click"=w522:bool)
        n306 = Unbundle By Name(w524) -> ("Row"=w518:i32)
        n307 = Greater Or Equal?(x=w518, y=0) -> (x >= y?=w523:bool)
        n308 = Index Array(array=w519, index (row)=w518) -> (element=w520:dbl[])  [unwired: 1 in]
        n309 = And(x=w522, y=w523) -> (x .and. y?=w521:bool)
        n310 = case shown="True" w521 {
          tunnel: w520 -> [_ w528]
          frame False {
          }
          frame True {
            n311 = To Long Integer(number=w528) -> (32bit integer=w527:i32[])
            n312 = for {
              tunnel: w527 -> [w529] mode=indexing
              i -> [w530]
              n313 = property on="GraphChart" class="WFGraph (strict)"("Active Cursor"=w530) -> (error out=w531:errorcluster)  [unwired: 2 in, 1 out]
              n314 = property on="GraphChart" class="WFGraph (strict)"(error in=w531, "Cursor.Cursor Index"=w529) -> ()  [unwired: 1 in, 2 out]
            }
          }
        }
      }
      event Timeout {
        n315 = event-data() -> ()  [unwired: 1 in, 1 out]
      }
    }
    n316 = Array To Spreadsheet String(array=w315, 3:"%g" ("format string")) -> (spreadsheet string=w374:string)  [unwired: 1 in]
    n317 = case shown="True" w375 {
      tunnel: [w653 w654] -> w373
      tunnel: "输入备注说明" -> [_ w663]
      tunnel: w374 -> [w653 w658]
      frame False {
      }
      frame True {
        n318 = Spreadsheet String To Array(delimiter (Tab)="\t", format string="%s", spreadsheet string=w658, array type (2D Dbl)=string[][] [] ("添加的数组")) -> (array=w659:string[][])
        n319 = for {
          tunnel: w659 -> [w673] mode=indexing
          tunnel: [w672] -> w657 mode=indexing
          tunnel: w663 -> [w667]
          i -> [w671]
          n320 = Not Equal?(x=0 ("y"), y=w671) -> (x != y?=w669:bool)
          n321 = Select(t="", s=w669, f=w667) -> (s? t:f=w668:string)
          n322 = Insert Into Array(array=w673, new element=w668) -> (w672:string[])  [unwired: 1 in]
        }
        n323 = flat-sequence {
          tunnel: w657 -> [w664]
          tunnel: [w664] -> w655
          frame #0 {
            n324 = local write "输入备注说明"("") -> ()
          }
        }
        n325 = Array To Spreadsheet String(array=w655, 3:"%s" ("format string")) -> (spreadsheet string=w654:string)  [unwired: 1 in]
      }
    }
    n326 = Write to Binary File(file (use dialog)=w392, data=w373, error in=w395, 5:FALSE ("预置数组或字符串大小？(T)")) -> (refnum out=w391:refnum<file>, error out=w394:errorcluster)  [unwired: 2 in, 1 out]
    n327 = Index Array(array=w262) -> (element #1=→"曲线0数字":dbl, element #2=→"曲线1数字":dbl, element #3=→"曲线2数字":dbl, element #4=→"曲线3数字":dbl, element #5=→"曲线4数字":dbl, element #6=→"曲线5数字":dbl)  [unwired: 6 in]
    n328 = case shown="True" "保存表格" {
      tunnel: w285 -> [_ w541]
      tunnel: w361 -> [_ w539]
      frame False {
      }
      frame True {
        n329 = Array To Spreadsheet String(array=w541, 3:"%s" ("格式字符串")) -> (spreadsheet string=w540:string)  [unwired: 1 in]
        n330 = File Dialog ("文件对话框")(6:"*.txt" ("类型（所有文件）"), 7:"请指定保存路径" ("提示"), 9:"临界安全表.txt" ("默认名称")) -> (0:w532:errorcluster, 1:w533:bool, 3:w534:path)  [unwired: 1 in, 4 out]
        n331 = Concatenate Strings(w540, w539) -> (w538:string)
        n332 = case shown="False" w533 {
          tunnel: w538 -> [w544 _]
          tunnel: w534 -> [w543 _]
          frame False {
            n333 = Open/Create/Replace File(file path (use dialog)=w543, operation (0:open)=T5."replace or create") -> (refnum out=w547:refnum<file>, error out=w549:errorcluster)  [unwired: 4 in, 1 out]
            n334 = Write to Text File(file (use dialog)=w547, text=w544, error in=w549) -> (refnum out=w546:refnum<file>, error out=w545:errorcluster)  [unwired: 1 in, 1 out]
            n335 = Close File(refnum=w546, error in=w545) -> ()  [unwired: 2 out]
          }
          frame True {
          }
        }
        n336 = call <vilib>:"Clear Errors.vi"("error in (no error)"=w532) -> ()  [unwired: 5 in, 2 out]
      }
    }
    n337 = Transpose 2D Array(2D array=w308) -> (transposed array=w309:dbl[][])
    n338 = Transpose 2D Array(2D array=w310) -> (transposed array=w311:dbl[][])
    n339 = for {
      tunnel: w311 -> [w459] mode=indexing
      tunnel: w309 -> [w460] mode=indexing
      shift-right: [w461] -> w307
      shift-left: dbl[][] [] -> [w463]
      # "交插通量与反应性"
      n340 = Build Array(w459, w460) -> (w462:dbl[][])
      n341 = Insert Into Array "数组插入"(array=w463, new element=w462) -> (w461:dbl[][])  [unwired: 2 in]
    }
    n342 = property on="保存表格" class="Bool"("DisabledEnum"=w332) -> ()  [unwired: 2 in, 2 out]
    n343 = Initialize Array(0.0 ("元素"), w277) -> (w281:dbl[])
    n344 = case shown="True" w363 {
      tunnel: w285 -> [_ w551]
      tunnel: w361 -> [_ w550]
      frame False {
      }
      frame True {
        n345 = property on="Table" class="Tbl (strict)"("Column Headers[]"=w551, "Col Headers Vis"=TRUE ("显示项:显示列首")) -> (error out=w553:errorcluster)  [unwired: 2 in, 1 out]
        n346 = Spreadsheet String To Array(format string="%s" ("格式字符串"), spreadsheet string=w550, array type (2D Dbl)=string[][] [] ("添加的数组")) -> (array=→"Table":string[][])  [unwired: 1 in]
        n347 = property on="Table" class="Tbl (strict)"(error in=w553, "Selection Size"=T6 {"Row"=0, "Column"=0} ("选择区域大小")) -> ()  [unwired: 1 in, 2 out]
      }
    }
    n348 = Reciprocal(x=w284) -> (1/x=w282:dbl[][])
    n349 = Insert Into Array(array=w282, new element=w281) -> (w274:dbl[][])  [unwired: 2 in]
    n350 = for {
      N: w277 -> [_]
      tunnel: w278 -> [w402]
      shift-right: [w400] -> w276
      shift-left: dbl[][] [] ("记录") -> [w403]
      i -> [w401]
      n351 = Insert Into Array(array=w403, index (col)=w401, new element=w402) -> (w400:dbl[][])  [unwired: 1 in]
    }
    n352 = Insert Into Array(array=w307, new element=w328) -> (w261:dbl[][])  [unwired: 2 in]
    n353 = Transpose 2D Array(2D array=w274) -> (transposed array=w269:dbl[][])
    n354 = flat-sequence {
      tunnel: w261 -> [w396]
      tunnel: [w396] -> w260
      tunnel: w260 -> [w397]
      frame #0 {
        n355 = invoke on="GraphChart" class="WFGraph (严格)" method="Reinit To Default"() -> ()  [unwired: 3 in, 3 out]
      }
      frame #1 {
        "GraphChart" <- w397
      }
    }
    n356 = global read "GlobalVariable.vi" "返回LOGO"() -> (w266:bool)
    n357 = local read "停止监督"() -> (w265:bool)
    n358 = Insert Into Array(array=w276, index (row)=w272, new element=w273) -> (w275:dbl[][])  [unwired: 1 in]
    n359 = Or(x=w265, y=w266) -> (x .or. y?=w264:bool)
    n360 = Transpose 2D Array(2D array=w275) -> (transposed array=w270:dbl[][])
    n361 = case shown="True" "显示临界曲线" {
      tunnel: w270 -> [_ w398]
      tunnel: w269 -> [_ w399]
      frame False {
      }
      frame True {
        n362 = call "XY_Dialog.vi"("Y输入"=w399, "X输入"=w398) -> ()  [unwired: 1 in]
      }
    }
  }
  n363 = while {
    tunnel: w111 -> [w750]
    tunnel: w109 -> [w726]
    tunnel: w108 -> [w725]
    stop <- w716 stop-if-true
    w748 = bool[] []  # 记录有无手动标尺
    # "显隐曲线并集合用到的标尺"
    n364 = call-poly <vilib>:"Acquire Input Data.vi"("device ID"=w725, "error in (no error)"=w726) -> ("button info"=w727:T9)  [unwired: 1 in, 16 out]
    n365 = Unbundle By Name(w727) -> ("button 1"=w724:bool, "button 2"=w723:bool, "button 3"=w722:bool, "button 4"=w721:bool)
    n366 = local read "GraphChart"() -> (w719:dbl[][])
    n367 = property on="X标尺最小-" class="Bool"("Visible"="自动/手动调整X标尺？") -> ()  [unwired: 2 in, 2 out]
    n368 = property on="X标尺最小+" class="Bool"("Visible"="自动/手动调整X标尺？") -> (error out=w742:errorcluster)  [unwired: 2 in, 1 out]
    n369 = Build Array("曲线开关0", "曲线开关1", "曲线开关2", "曲线开关3", "曲线开关4", "曲线开关5") -> (w756:bool[])
    n370 = Compound Arithmetic op=OR(w724, w723, w722, w721) -> (w720:bool)
    n371 = case shown="False" w720 {
      frame False {
        n372 = Wait Until Next ms Multiple(millisecond multiple=u32 1000) -> ()  [unwired: 1 out]
      }
      frame True {
        n373 = Wait Until Next ms Multiple(millisecond multiple=u32 100) -> ()  [unwired: 1 out]
      }
    }
    n374 = Array Size(array=w719) -> (size(s)=w740:i32[])
    n375 = property on="GraphChart" class="WFGraph (strict)"(error in=w742, "ActXScl"=0 ("活动X标尺")) -> (error out=w737:errorcluster)  [unwired: 1 in, 1 out]
    n376 = for {
      tunnel: w756 -> [w984] mode=indexing
      tunnel: w750 -> [w982] mode=indexing
      shift-right: [w981] -> w753
      shift-left: i32[] [] ("添加的数组") -> [w983]
      shift-right: [w978] -> w751
      shift-left: i32[] [] ("添加的数组") -> [w980]
      i -> [w979]
      n377 = case shown="True" w984 {
        tunnel: w983 -> [w986 w992]
        tunnel: w982 -> [_ w991]
        tunnel: [w986 w990] -> w981
        tunnel: w980 -> [w985 w989]
        tunnel: w979 -> [_ w988]
        tunnel: [w985 w987] -> w978
        frame False {
        }
        frame True {
          n378 = Insert Into Array(array=w989, new element=w988) -> (w987:i32[])  [unwired: 1 in]
          n379 = Insert Into Array(array=w992, new element=w991) -> (w990:i32[])  [unwired: 1 in]
        }
      }
      n380 = property on="GraphChart" class="WFGraph (strict)"("Active Plot"=w979, "Plot.Visible?"=w984) -> ()  [unwired: 2 in, 2 out]
    }
    n381 = Index Array(array=w740, index=1 ("索引")) -> (element=w738:i32)
    n382 = property on="GraphChart" class="WFGraph (strict)"(error in=w737) -> (error out=w736:errorcluster, "XScale.Maximum"=w734:dbl)  [unwired: 1 in, 1 out]
    n383 = for {
      N: 8 -> [_]
      tunnel: w753 -> [w821]
      tunnel: w751 -> [w822]
      tunnel: w719 -> [w820]
      tunnel: "自动调整Y标尺？" -> [w818]
      shift-right: [w816] -> w747
      shift-left: w748 -> [w817]
      i -> [w823]
      # "根据标尺有无被用到决定是否显示标尺"
      n384 = for {
        tunnel: w821 -> [w977] mode=indexing
        tunnel: w823 -> [w976]
        tunnel: [w975] -> w824
        stop <- w975 stop-if-true
        n385 = Equal?(x=w977, y=w976) -> (x = y?=w975:bool)
      }
      n386 = property on="GraphChart" class="WFGraph (strict)"("ActYScl"=w823) -> (error out=w825:errorcluster)  [unwired: 2 in, 1 out]
      n387 = property on="GraphChart" class="WFGraph (strict)"(error in=w825, "YScale.Visible"=w824) -> (error out=w819:errorcluster)  [unwired: 1 in, 1 out]
      n388 = case shown="True" w824 {
        tunnel: w823 -> [_ w844]
        tunnel: w822 -> [_ w843]
        tunnel: w821 -> [_ w845]
        tunnel: w820 -> [_ w842]
        tunnel: w819 -> [_ w834]
        tunnel: w818 -> [_ w832]
        tunnel: w817 -> [w826 w829]
        tunnel: [w826 w828] -> w816
        frame False {
        }
        frame True {
          n389 = property on="GraphChart" class="WFGraph (strict)"(error in=w834) -> (error out=w836:errorcluster, "YScale.ScaleFit"=w839:u8)  [unwired: 1 in, 1 out]
          n390 = property on="GraphChart" class="WFGraph (strict)"(error in=w834) -> ("YScale.Increment"=w833:dbl)  [unwired: 1 in, 2 out]
          n391 = for {
            tunnel: w845 -> [w955] mode=indexing
            tunnel: w844 -> [w954]
            tunnel: w843 -> [w953]
            tunnel: w842 -> [w950]
            shift-right: [w947] -> w835
            shift-left: inf -> [w949]
            shift-right: [w946] -> w837
            shift-left: -inf -> [w948]
            i -> [w952]
            # "正在显示的标尺则考虑调整"
            n392 = Equal?(x=w955, y=w954) -> (x = y?=w951:bool)
            n393 = case shown="True" w951 {
              tunnel: w953 -> [_ w970]
              tunnel: w952 -> [_ w969]
              tunnel: w950 -> [_ w968]
              tunnel: [w957 w961] -> w947
              tunnel: w949 -> [w957 w960]
              tunnel: w948 -> [w956 w964]
              tunnel: [w956 w963] -> w946
              frame False {
              }
              frame True {
                n394 = Index Array(array=w970, index=w969) -> (element=w967:i32)
                n395 = Index Array(array=w968, index (row)=w967) -> (element=w966:dbl[])  [unwired: 1 in]
                n396 = Array Max & Min(array=w966) -> (max value=w962:dbl, min value=w959:dbl)  [unwired: 2 out]
                n397 = Greater?(x=w962, y=w964) -> (0:w965:bool)
                n398 = Less?(x=w959, y=w960) -> (x < y?=w958:bool)
                n399 = case shown="False" w965 {
                  tunnel: w964 -> [w973 _]
                  tunnel: [w973 w974] -> w963
                  tunnel: w962 -> [_ w974]
                  frame False {
                  }
                  frame True {
                  }
                }
                n400 = case shown="True" w958 {
                  tunnel: w960 -> [w971 _]
                  tunnel: [w971 w972] -> w961
                  tunnel: w959 -> [_ w972]
                  frame False {
                  }
                  frame True {
                  }
                }
              }
            }
          }
          n401 = Equal?(x=w839, y=u8 0) -> (x = y?=w830:bool)
          n402 = case shown="True" w830 {
            selector: w830 -> [w863 _]
            tunnel: w837 -> [_ w874]
            tunnel: w836 -> [w862 w885]
            tunnel: w835 -> [_ w869]
            tunnel: w830 -> [_ _]
            tunnel: w833 -> [_ w866]
            tunnel: [w862 w865] -> w831
            tunnel: [w863 w864] -> w827
            tunnel: w830 -> [_ w864]
            frame False {
            }
            frame True {
              n403 = property on="GraphChart" class="WFGraph (strict)"(error in=w885) -> (error out=w883:errorcluster, "YScale.Maximum"=w884:dbl)  [unwired: 1 in, 1 out]
              n404 = property on="GraphChart" class="WFGraph (strict)"(error in=w885) -> (error out=w875:errorcluster, "YScale.Minimum"=w876:dbl)  [unwired: 1 in, 1 out]
              n405 = case shown="True" "Y标尺最小+" {
                tunnel: w874 -> [_ w909]
                tunnel: w876 -> [w901 w907]
                tunnel: w875 -> [w902 w906]
                tunnel: [w902 w905] -> w872
                tunnel: [w901 w904] -> w870
                tunnel: w866 -> [_ w903]
                frame False {
                }
                frame True {
                  n406 = Greater?(x=w907, y=w909) -> (0:w908:bool)
                  n407 = case shown="True" w908 {
                    tunnel: [w911 w915] -> w904
                    tunnel: w909 -> [_ w915]
                    tunnel: w907 -> [w912 _]
                    tunnel: w906 -> [w913 w914]
                    tunnel: [w913 w914] -> w905
                    tunnel: w903 -> [w910 _]
                    frame False {
                      n408 = Add(x=w912, y=w910) -> (x+y=w911:dbl)
                    }
                    frame True {
                    }
                  }
                }
              }
              n409 = case shown="True" "Y标尺最大+" {
                tunnel: w874 -> [_ w939]
                tunnel: w884 -> [w931 w937]
                tunnel: w883 -> [w932 w936]
                tunnel: [w932 w935] -> w880
                tunnel: [w931 w934] -> w879
                tunnel: w866 -> [_ w933]
                frame False {
                }
                frame True {
                  n410 = Greater?(x=w937, y=w939) -> (0:w938:bool)
                  n411 = case shown="False" w938 {
                    tunnel: [w941 w945] -> w934
                    tunnel: w939 -> [_ w945]
                    tunnel: w937 -> [w942 _]
                    tunnel: w936 -> [w943 w944]
                    tunnel: [w943 w944] -> w935
                    tunnel: w933 -> [w940 _]
                    frame False {
                      n412 = Add(x=w942, y=w940) -> (x+y=w941:dbl)
                    }
                    frame True {
                    }
                  }
                }
              }
              n413 = case shown="True" "Y标尺最大-" {
                tunnel: w869 -> [_ w924]
                tunnel: w879 -> [w917 w922]
                tunnel: w880 -> [w916 w921]
                tunnel: [w917 w920] -> w878
                tunnel: [w916 w919] -> w877
                tunnel: w866 -> [_ w918]
                frame False {
                }
                frame True {
                  n414 = Less?(x=w922, y=w924) -> (x < y?=w923:bool)
                  n415 = case shown="False" w923 {
                    tunnel: [w926 w930] -> w920
                    tunnel: w924 -> [_ w930]
                    tunnel: w922 -> [w927 _]
                    tunnel: w921 -> [w928 w929]
                    tunnel: [w928 w929] -> w919
                    tunnel: w918 -> [w925 _]
                    frame False {
                      n416 = Subtract(x=w927, y=w925) -> (x-y=w926:dbl)
                    }
                    frame True {
                    }
                  }
                }
              }
              n417 = case shown="True" "Y标尺最小-" {
                tunnel: w869 -> [_ w894]
                tunnel: w870 -> [w887 w892]
                tunnel: w872 -> [w886 w891]
                tunnel: [w887 w890] -> w867
                tunnel: [w886 w889] -> w868
                tunnel: w866 -> [_ w888]
                frame False {
                }
                frame True {
                  n418 = Less?(x=w892, y=w894) -> (x < y?=w893:bool)
                  n419 = case shown="False" w893 {
                    tunnel: [w896 w900] -> w890
                    tunnel: w894 -> [_ w900]
                    tunnel: w892 -> [w897 _]
                    tunnel: w891 -> [w898 w899]
                    tunnel: [w898 w899] -> w889
                    tunnel: w888 -> [w895 _]
                    frame False {
                      n420 = Subtract(x=w897, y=w895) -> (x-y=w896:dbl)
                    }
                    frame True {
                    }
                  }
                }
              }
              n421 = property on="GraphChart" class="WFGraph (strict)"(error in=w877, "YScale.Maximum"=w878) -> (error out=w865:errorcluster)  [unwired: 1 in, 1 out]
              n422 = property on="GraphChart" class="WFGraph (strict)"(error in=w868, "YScale.Minimum"=w867) -> ()  [unwired: 1 in, 2 out]
            }
          }
          n423 = case shown="True" w832 {
            tunnel: w831 -> [_ w854]
            tunnel: w827 -> [_ w853]
            frame False {
            }
            frame True {
              n424 = property on="GraphChart" class="WFGraph (strict)"(error in=w854) -> (error out=w852:errorcluster, "YScale.NameLbl.Text"=w855:string)  [unwired: 1 in, 1 out]
              n425 = Select(t="-手动调整转为自动调整？" ("format string"), s=w853, f="-自动调整转为手动调整？" ("format string")) -> (s? t:f=w856:string)
              n426 = Concatenate Strings ("连接字符串")(w855, w856) -> (w848:string)
              n427 = Two Button Dialog(message=w848, 1:"否" ("F按钮名称（“取消”）"), 2:"是" ("T按钮名称（“确定”）")) -> (T button?=w849:bool)
              n428 = case shown="True" w849 {
                tunnel: w853 -> [_ w861]
                tunnel: w852 -> [_ w857]
                frame False {
                }
                frame True {
                  n429 = Select(t=u8 2 ("y"), s=w861, f=u8 0 ("y")) -> (s? t:f=w858:u8)
                  n430 = property on="GraphChart" class="WFGraph (strict)"(error in=w857, "YScale.ScaleFit"=w858) -> ()  [unwired: 1 in, 2 out]
                }
              }
            }
          }
          n431 = Insert Into Array(array=w829, new element=w827) -> (w828:bool[])  [unwired: 1 in]
        }
      }
    }
    n432 = property on="GraphChart" class="WFGraph (strict)"(error in=w736) -> (error out=w735:errorcluster, "XScale.Minimum"=w733:dbl)  [unwired: 1 in, 1 out]
    n433 = Subtract(x=w734, y=w733) -> (x-y=w732:dbl)
    n434 = Multiply(x=w732, y=0.1) -> (x*y=w730:dbl)
    n435 = Round Toward +Infinity(x=w730) -> (ceil(x): smallest int >= x=w729:dbl)
    n436 = case shown="True" "自动/手动调整X标尺？" {
      tunnel: [2 ("活动X标尺") 0 ("活动X标尺")] -> w743
      tunnel: [w787 w789] -> w741
      tunnel: w735 -> [w787 w800]
      tunnel: w738 -> [_ w805]
      tunnel: w733 -> [_ w799]
      tunnel: w729 -> [_ w791]
      frame False {
      }
      frame True {
        n437 = Subtract(x=w805, y=10.0) -> (x-y=w798:dbl)
        n438 = Subtract(x=w798, y=w791) -> (x-y=w797:dbl)
        n439 = Less?(x=w799, y=w797) -> (x < y?=w802:bool)
        n440 = And(x="X标尺最小+", y=w802) -> (x .and. y?=w804:bool)
        n441 = case shown="True" w804 {
          tunnel: w799 -> [w812 w815]
          tunnel: [w812 w814] -> w793
          tunnel: w791 -> [_ w813]
          frame False {
          }
          frame True {
            n442 = Add(x=w815, y=w813) -> (x+y=w814:dbl)
          }
        }
        n443 = Add(x=10.0, y=w791) -> (x+y=w790:dbl)
        n444 = Greater?(x=w793, y=w790) -> (0:w794:bool)
        n445 = And(x="X标尺最小-", y=w794) -> (x .and. y?=w796:bool)
        n446 = case shown="True" w796 {
          tunnel: w793 -> [w808 w811]
          tunnel: [w808 w810] -> w801
          tunnel: w791 -> [_ w809]
          frame False {
          }
          frame True {
            n447 = Subtract(x=w811, y=w809) -> (x-y=w810:dbl)
          }
        }
        n448 = property on="GraphChart" class="WFGraph (strict)"(error in=w800, "XScale.Minimum"=w801) -> (error out=w789:errorcluster)  [unwired: 1 in, 1 out]
      }
    }
    n449 = property on="GraphChart" class="WFGraph (strict)"(error in=w741, "XScale.ScaleFit"=w743) -> ()  [unwired: 1 in, 2 out]
    n450 = for {
      N: 6 -> [_]
      i -> [w765]
      # "数值显示颜色同步于曲线"
      n451 = property on="GraphChart" class="WFGraph (strict)"("Active Plot"=w765) -> (error out=w768:errorcluster)  [unwired: 2 in, 1 out]
      n452 = property on="GraphChart" class="WFGraph (strict)"(error in=w768) -> (error out=w767:errorcluster, "Plot.Plot Color"=w766:u32)  [unwired: 1 in, 1 out]
      n453 = case shown="5" w765 {
        tunnel: w767 -> [w770 w773 w776 w779 w782 w785]
        tunnel: w766 -> [w769 w772 w775 w778 w781 w784]
        frame 1 {
          n454 = property on="曲线1数字" class="DigNum (strict)"(error in=w770, "Caption.TextColor"=w769) -> (error out=w771:errorcluster)  [unwired: 1 in, 1 out]
          n455 = property on="曲线1数字" class="DigNum (strict)"(error in=w771, "NumText.TextColor"=w769) -> ()  [unwired: 1 in, 2 out]
        }
        frame 2 {
          n456 = property on="曲线2数字" class="DigNum (strict)"(error in=w773, "Caption.TextColor"=w772) -> (error out=w774:errorcluster)  [unwired: 1 in, 1 out]
          n457 = property on="曲线2数字" class="DigNum (strict)"(error in=w774, "NumText.TextColor"=w772) -> ()  [unwired: 1 in, 2 out]
        }
        frame 3 {
          n458 = property on="曲线3数字" class="DigNum (strict)"(error in=w776, "Caption.TextColor"=w775) -> (error out=w777:errorcluster)  [unwired: 1 in, 1 out]
          n459 = property on="曲线3数字" class="DigNum (strict)"(error in=w777, "NumText.TextColor"=w775) -> ()  [unwired: 1 in, 2 out]
        }
        frame 4 {
          n460 = property on="曲线4数字" class="DigNum (strict)"(error in=w779, "Caption.TextColor"=w778) -> (error out=w780:errorcluster)  [unwired: 1 in, 1 out]
          n461 = property on="曲线4数字" class="DigNum (strict)"(error in=w780, "NumText.TextColor"=w778) -> ()  [unwired: 1 in, 2 out]
        }
        frame 5 {
          n462 = property on="曲线5数字" class="DigNum (strict)"(error in=w782, "Caption.TextColor"=w781) -> (error out=w783:errorcluster)  [unwired: 1 in, 1 out]
          n463 = property on="曲线5数字" class="DigNum (strict)"(error in=w783, "NumText.TextColor"=w781) -> ()  [unwired: 1 in, 2 out]
        }
        frame 0, Default {
          n464 = property on="曲线0数字" class="DigNum (strict)"(error in=w785, "Caption.TextColor"=w784) -> (error out=w786:errorcluster)  [unwired: 1 in, 1 out]
          n465 = property on="曲线0数字" class="DigNum (strict)"(error in=w786, "NumText.TextColor"=w784) -> ()  [unwired: 1 in, 2 out]
        }
      }
    }
    n466 = Or Array Elements(Boolean array=w747) -> (logical OR=w746:bool)
    n467 = global read "GlobalVariable.vi" "返回LOGO"() -> (w717:bool)
    n468 = property on="Y标尺最小-" class="Bool"("Visible"=w746) -> ()  [unwired: 2 in, 2 out]
    n469 = property on="Y标尺最小+" class="Bool"("Visible"=w746) -> ()  [unwired: 2 in, 2 out]
    n470 = property on="Y标尺最大+" class="Bool"("Visible"=w746) -> ()  [unwired: 2 in, 2 out]
    n471 = property on="Y标尺最大-" class="Bool"("Visible"=w746) -> ()  [unwired: 2 in, 2 out]
    n472 = Or(x="停止监督", y=w717) -> (x .or. y?=w716:bool)
  }
  n473 = case shown="True" w119 {
    tunnel: [FALSE ("返回LOGO") FALSE ("返回LOGO")] -> w21
    frame False {
    }
    frame True {
      n474 = global write "GlobalVariable.vi" "有无接收"(FALSE ("写完毕")) -> ()
      n475 = local write "停止监督"(FALSE ("Exit")) -> ()
      n476 = global write "GlobalVariable.vi" "子VI退出"(TRUE ("子VI退出")) -> ()
    }
  }
  n477 = flat-sequence {
    tunnel: w116 -> [w1003]
    tunnel: w112 -> [w1004]
    tunnel: w49 -> [w1002]
    tunnel: [w1004] -> w40
    tunnel: [w1003] -> w39
    tunnel: [w998] -> w43
    frame #0 {
      n478 = Get Date/Time String(date format (0)=enum16{"short", "long", "abbreviated"}."long" ("日期格式(0)"), want seconds? (F)=TRUE ("需要秒？(F)")) -> (date string=w1007:string, time string=w1006:string)  [unwired: 1 in]
      n479 = call <vilib>:"Space Constant.vi"() -> ("String"=w1005:string)
      n480 = Concatenate Strings "连接字符串"(w1007, w1005, w1006) -> (w999:string)
      n481 = Insert Into Array(array=w1002, new element="结束时间：" ("字符串")) -> (w1000:string[])  [unwired: 1 in]
      n482 = Insert Into Array(array=w1000, new element=w999) -> (w998:string[])  [unwired: 1 in]
    }
  }
  n483 = global write "GlobalVariable.vi" "返回LOGO"(w21) -> ()
  n484 = Array To Spreadsheet String(array=w43, 3:"%s" ("format string")) -> (spreadsheet string=w38:string)  [unwired: 1 in]
  n485 = Write to Binary File(file (use dialog)=w40, data=w38, error in=w39, 5:FALSE ("预置数组或字符串大小？(T)")) -> (refnum out=w42:refnum<file>, error out=w41:errorcluster)  [unwired: 2 in, 1 out]
  n486 = Close File(refnum=w42, error in=w41) -> (error out=w48:errorcluster)  [unwired: 1 out]
  n487 = call <vilib>:"Simple Error Handler.vi"("error in (no error)"=w48) -> ()  [unwired: 4 in, 5 out]
